vi "HexToBinary.vi"(0 "Hex String":string, 1 "error in":errorcluster) -> (2 "output string":string, 3 "Value":dbl format="%.2f", 4 "Bits displayed":u32, 5 "error out":errorcluster)   [LabVIEW 2014]
doc: "Convert a hex string of any length to a binary string. Generates Error Out if invalid hex character is entered."
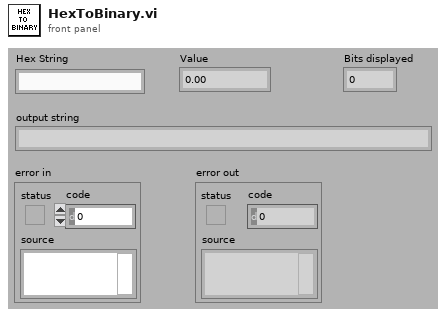
[diagram p1: front panel]
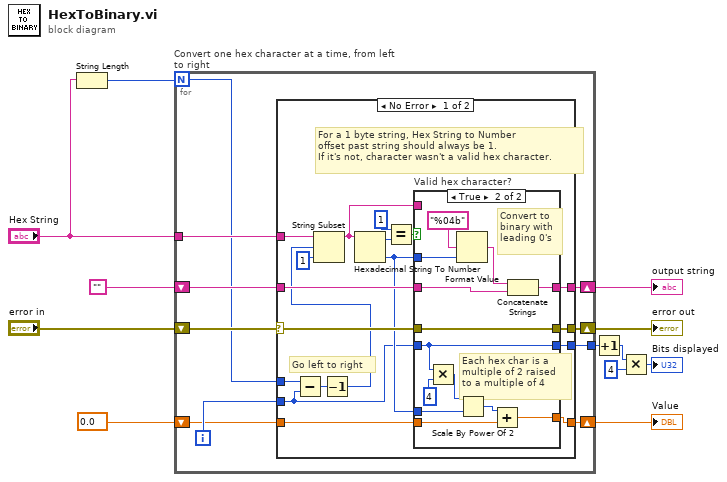
[diagram p0: block diagram]
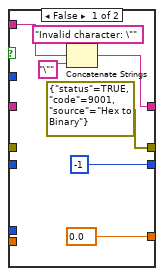
[diagram p2: hidden frame]
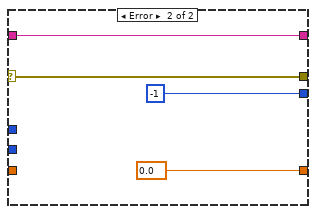
[diagram p3: hidden frame]
diagram:
  n1 = String Length(string="Hex String") -> (length=w9:i32)
  n2 = for "Convert one hex character at a time, from left to right" {
    N: w9 -> [w13]
    tunnel: "Hex String" -> [w22]
    shift-right: [w21] -> w11
    shift-left: "" -> [w20]
    shift-right: [w18] -> w7
    shift-left: "error in" -> [w17]
    tunnel: [w16] -> w6
    shift-right: [w14] -> w1
    shift-left: 0.0 -> [w15]
    i -> [w19]
    n3 = case shown="No Error" w17 {
      selector: w17 -> [w32 w64]
      tunnel: w22 -> [w39 _]
      tunnel: [w38 w63] -> w21
      tunnel: w20 -> [w37 w63]
      tunnel: w19 -> [w23 _]
      tunnel: [w34 w64] -> w18
      tunnel: [w31 -1] -> w16
      tunnel: w15 -> [w30 _]
      tunnel: [w29 0.0] -> w14
      tunnel: w13 -> [w26 _]
      frame No Error {
        # "Go left to right"
        # "For a 1 byte string, Hex String to Number\noffset past string should always be 1.\nIf it's not, character wasn't a valid hex character."
        n4 = Subtract(x=w26, y=w23) -> (x-y=w25:i32)
        n5 = Decrement(x=w25) -> (x-1=w24:i32)
        n6 = String Subset(string=w39, offset (0)=w24, length (rest)=1 ("length (rest)")) -> (substring=w33:string)
        n7 = Hexadecimal String To Number(string=w33) -> (offset past number=w28:i32, number=w27:u32)  [unwired: 2 in]
        n8 = Equal?(x=1, y=w28) -> (x = y?=w35:bool)
        n9 = case "Valid hex character?" shown="True" w35 {
          tunnel: [w46 w60] -> w38
          tunnel: w27 -> [_ w59]
          tunnel: w37 -> [_ w48]
          tunnel: [errorcluster {"status"=TRUE, "code"=9001, "source"="Hex to Binary"} ("error in (no error)") w57] -> w34
          tunnel: w32 -> [_ w57]
          tunnel: w33 -> [w44 _]
          tunnel: w23 -> [_ w53]
          tunnel: [-1 w53] -> w31
          tunnel: w27 -> [_ w54]
          tunnel: w30 -> [_ w56]
          tunnel: [0.0 w55] -> w29
          frame False {
            n10 = Concatenate Strings("Invalid character: \"", w44, "\"" ("string")) -> (w46:string)
          }
          frame True {
            # "Each hex char is a\nmultiple of 2 raised\nto a multiple of 4"
            # "Convert to\nbinary with\nleading 0's"
            n11 = Multiply(x=w53, y=4) -> (x*y=w51:i32)
            n12 = Format Value(format string="%04b", value (0)=w59) -> (output string=w49:string)  [unwired: 1 in]
            n13 = Scale By Power Of 2(n=w51, x=w54) -> (x*2^n=w50:u32)
            n14 = Add(x=w50, y=w56) -> (x+y=w55:dbl)
            n15 = Concatenate Strings(w49, w48) -> (w60:string)
          }
        }
      }
      frame Error {
      }
    }
  }
  "output string" <- w11
  "error out" <- w7
  "Value" <- w1
  n16 = Increment(x=w6) -> (x+1=w3:i32)
  n17 = Multiply(x=w3, y=4) -> (x*y=→"Bits displayed":i32)
